vi "Register Events.vi"(8 "error in (no error)":errorcluster, 11 "Execution API In":refnum<class "Execution API.lvclass">) -> (0 "error out":errorcluster, 2 "Result Events":T1, 3 "Execution API Out":refnum<class "Execution API.lvclass">)   [LabVIEW 2020, in "Execution API.lvclass"]
uses:
  Execution API.lvclass
  Result Classes/Method Result/Method Result.lvclass
  Result Classes/Test Case Result/Test Case Result.lvclass
  Result Classes/Test Suite Result/Test Suite Result.lvclass
  Execution API.lvclass/Execution API.ctl
  Result Collector/Result Collector.lvclass
  Test Runner/Test Runner.lvclass
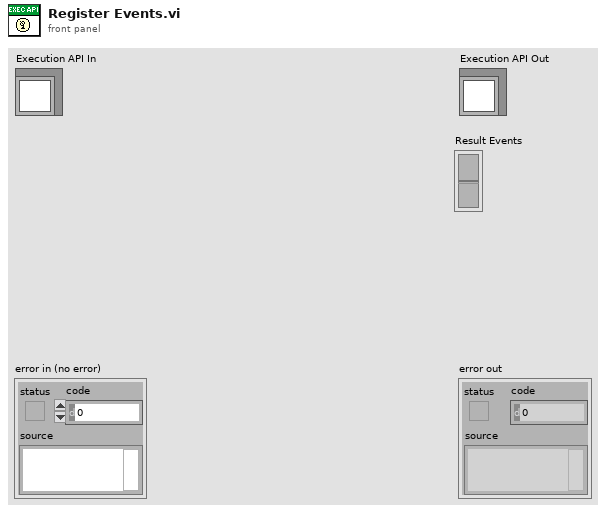
[diagram p1: front panel]
types:
  T1 = cluster{"Event Registration Refnum":refnum<event-registration>, "Event Registration Refnum":refnum<event-registration>}
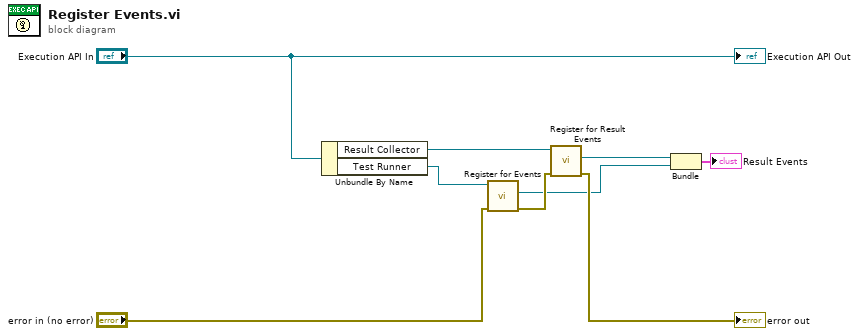
[diagram p0: block diagram]
diagram:
  n1 = Unbundle By Name("Execution API In") -> ("Result Collector"=w8:refnum<class "Result Collector.lvclass">, "Test Runner"=w7:refnum<class "Test Runner.lvclass">)
  n2 = call "Register for Events.vi"("error in (no error)"="error in (no error)", "Test Runner In"=w7) -> ("error out"=w6:errorcluster, "Event Registration Refnum"=w3:refnum<event-registration>)  [unwired: 7 in, 1 out]
  n3 = call "Register for Result Events.vi"("error in (no error)"=w6, "Result Collector In"=w8) -> ("error out"=→"error out":errorcluster, "Event Registration Refnum"=w2:refnum<event-registration>)  [unwired: 7 in, 1 out]
  n4 = Bundle("Event Registration Refnum"=w2, "Event Registration Refnum"=w3) -> (→"Result Events":T1)  [unwired: 1 in]
  "Execution API Out" <- "Execution API In"
